vi "5 Sync - TSN Magicness.vi"() -> ()   [LabVIEW 2023]
doc: "This example demonstrates how to acquire a single buffer of voltage measurements using a DAQmx device.\n\nFor instructions on how to connect your signals to the DAQ device, refer to your device documentation."
uses:
  <resource>/objmgr/daqmx.rc
  <vilib>/DAQmx/create/channels.llb/DAQmx Create Channel (AI-Voltage-Basic).vi
  <vilib>/DAQmx/create/channels.llb/DAQmx Create Channel (CO-Pulse Generation-Frequency).vi
  <vilib>/DAQmx/configure/timing.llb/DAQmx Timing (Implicit).vi
  <vilib>/DAQmx/configure/timing.llb/DAQmx Timing (Sample Clock).vi
  <vilib>/DAQmx/read.llb/DAQmx Read (Analog 1D Wfm NChan NSamp).vi
panel:
  in  "stop":bool
  in  "Square Wave Output: Terminal":tag="/MIODAQ/PFI0"
  in  "Square Wave Output: Source":tag="MIODAQ/ctr0"
  out "Skew":dbl=-1.072865529480623
  out "Waveform Graph":waveform(dbl)[](graph)=[{"t0"=timestamp(3851425488.627929 s since 1904-01-01), "dt"=9.999999999999972e-06, "Y"=array[100000 elements], "attributes"=variant("NI_ChannelName"=variant(string "MIODAQ/ai0"), "NI_UnitDescription"=variant(string "Volts"))}, {"t0"=timestamp(3851425488.628186 s since 1904-01-01), "dt"=9.999999999999972e-06, "Y"=array[100000 elements], "attributes"=variant("NI_ChannelName"=variant(string "cDAQ9189-2628AACMod1/ai0"), "NI_UnitDescription"=variant(string "Volts"))}]
  in  "Device 1 & 2: Sample Rate":dbl=100000.0
  in  "Device 1 & 2: Sample Clock Source":tag="OnboardClock"
  in  "Device 1 & 2: Analog Input Channel":tag="cDAQ9189-2628AACMod1/ai0, cDAQ9189-2628AD1Mod1/ai0"
  # "Channel Settings"
  # "Acquired Data"
  # "Timing Settings"
  # "Output Signal Settings"
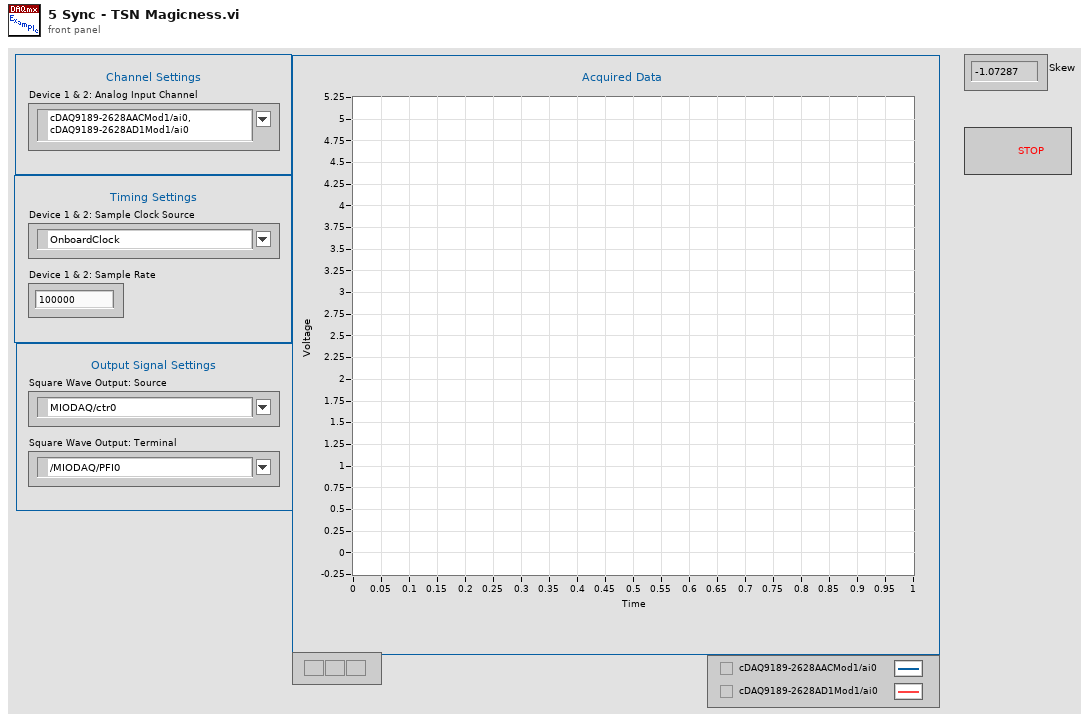
[diagram p1: front panel]
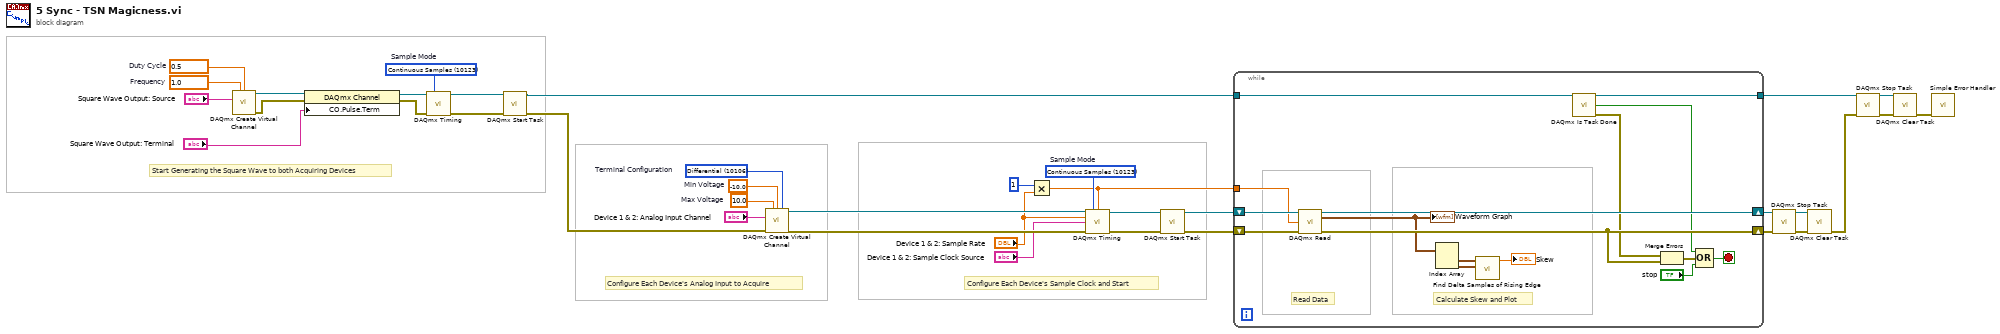
[diagram p0: block diagram]
diagram:
  w18 = 10.0  # Max Voltage
  w19 = -10.0  # Min Voltage
  w20 = 10106 items=["default"=-1, "RSE"=10083, "NRSE"=10078, "Differential"=10106, "Pseudodifferential"=12529]  # Terminal Configuration
  w13 = 10123 items=["Finite Samples"=10178, "Continuous Samples"=10123, "Hardware Timed Single Point"=12522]  # Sample Mode
  w34 = 1.0  # Frequency
  w35 = 0.5  # Duty Cycle
  w27 = 10123 items=["Finite Samples"=10178, "Continuous Samples"=10123, "Hardware Timed Single Point"=12522]  # Sample Mode
  # "Configure Each Device's Sample Clock and Start"
  # "Configure Each Device's Analog Input to Acquire"
  # "Start Generating the Square Wave to both Acquiring Devices"
  n1 = call-poly <vilib>:"DAQmx Create Virtual Channel.vi"("frequency"=w34, "duty cycle"=w35, "counter"="Square Wave Output: Source") -> ("task out"=w29:refnum<k21>, "error out"=w30:errorcluster)  [unwired: 11 in]
  n2 = property class="DAQmx Channel"(reference=w29, error in=w30, "CO.Pulse.Term"="Square Wave Output: Terminal") -> (reference out=w33:refnum<k21>, error out=w32:errorcluster)
  n3 = call-poly <vilib>:"DAQmx Timing.vi"("task/channels in"=w33, "sample mode"=w27, "error in"=w32) -> ("task out"=w37:refnum<k21>, "error out"=w36:errorcluster)  [unwired: 11 in]
  n4 = call <vilib>:"DAQmx Start Task.vi"("task/channels in"=w37, "error in"=w36) -> ("task out"=w7:refnum<k21>, "error out"=w5:errorcluster)  [unwired: 12 in]
  n5 = call-poly <vilib>:"DAQmx Create Virtual Channel.vi"("maximum value"=w18, "minimum value"=w19, "input terminal configuration"=w20, "physical channels"="Device 1 & 2: Analog Input Channel", "error in"=w5) -> ("task out"=w23:refnum<k21>, "error out"=w24:errorcluster)  [unwired: 9 in]
  n6 = Multiply(x=1, y="Device 1 & 2: Sample Rate") -> (x*y=w8:dbl)
  n7 = call-poly <vilib>:"DAQmx Timing.vi"("task/channels in"=w23, "sample mode"=w13, "samples per channel"=w8, "rate"="Device 1 & 2: Sample Rate", "source"="Device 1 & 2: Sample Clock Source", "error in"=w24) -> ("task out"=w3:refnum<k21>, "error out"=w4:errorcluster)  [unwired: 8 in]
  n8 = call <vilib>:"DAQmx Start Task.vi"("task/channels in"=w3, "error in"=w4) -> ("task out"=w22:refnum<k21>, "error out"=w9:errorcluster)  [unwired: 12 in]
  n9 = while {
    shift-right: [w51] -> w15
    shift-left: w22 -> [w52]
    shift-right: [w48] -> w12
    shift-left: w9 -> [w50]
    tunnel: w8 -> [w49]
    tunnel: w7 -> [w44]
    tunnel: [w41] -> w6
    stop <- w45 stop-if-true
    # "Read Data"
    # "Calculate Skew and Plot"
    n10 = call-poly <vilib>:"DAQmx Read.vi"("task/channels in"=w52, "number of samples per channel"=w49, "error in"=w50) -> ("task out"=w51:refnum<k21>, "data"=w40:waveform(dbl)[], "error out"=w48:errorcluster)  [unwired: 10 in]
    "Waveform Graph" <- w40
    n11 = Index Array(array=w40) -> (element #1=w39:waveform(dbl), element #2=w38:waveform(dbl))  [unwired: 2 in]
    n12 = call "Find Delta Samples of Rising Edge.vi"("Channel 2"=w38, "Channel 1"=w39) -> ("Sample Offset"=→"Skew":dbl)  [unwired: 9 in]
    n13 = call <vilib>:"DAQmx Is Task Done.vi"("task/channels in"=w44) -> ("task out"=w41:refnum<k21>, "task done?"=w42:bool, "error out"=w43:errorcluster)  [unwired: 12 in]
    n14 = Merge Errors(w43, w48) -> (w47:errorcluster)
    n15 = Compound Arithmetic op=OR(w42, w47, "stop") -> (w45:bool)
  }
  n16 = call <vilib>:"DAQmx Stop Task.vi"("task/channels in"=w15, "error in"=w12) -> ("task out"=w17:refnum<k21>, "error out"=w16:errorcluster)  [unwired: 12 in]
  n17 = call <vilib>:"DAQmx Clear Task.vi"("task in"=w17, "error in"=w16) -> ("error out"=w1:errorcluster)  [unwired: 13 in]
  n18 = call <vilib>:"DAQmx Stop Task.vi"("task/channels in"=w6, "error in"=w1) -> ("task out"=w25:refnum<k21>, "error out"=w26:errorcluster)  [unwired: 12 in]
  n19 = call <vilib>:"DAQmx Clear Task.vi"("task in"=w25, "error in"=w26) -> ("error out"=w2:errorcluster)  [unwired: 13 in]
  n20 = call <vilib>:"Simple Error Handler.vi"("error in (no error)"=w2) -> ()  [unwired: 4 in, 5 out]
